vi "xy_graph_coil.vi"() -> ()   [LabVIEW 2019]
panel:
  out "XY Graph":cluster{dbl[], dbl[]}(graph)
  in  "stop":bool
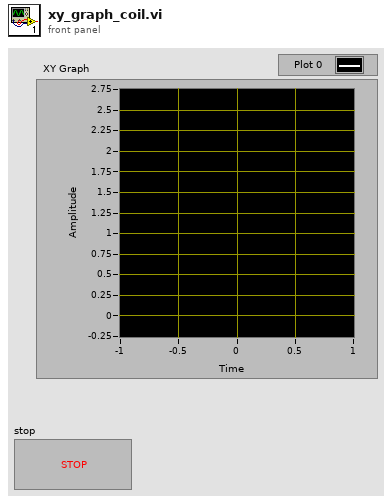
[diagram p1: front panel]
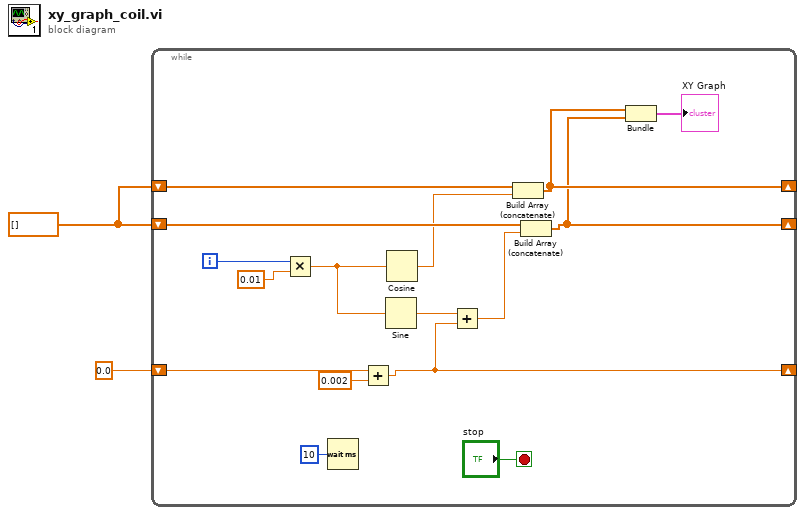
[diagram p0: block diagram]
diagram:
  w2 = dbl[] []
  n1 = while {
    shift-right: [w12] -> _
    shift-left: w2 -> [w16]
    shift-right: [w13] -> _
    shift-left: w2 -> [w15]
    shift-right: [w3] -> _
    shift-left: 0.0 -> [w7]
    i -> [w11]
    stop <- "stop" stop-if-true
    n2 = Multiply(x=w11, y=0.01) -> (x*y=w9:dbl)
    n3 = Wait (ms)(milliseconds to wait=u32 10) -> ()  [unwired: 1 out]
    n4 = Add(x=w7, y=0.002) -> (x+y=w3:dbl)
    n5 = Sine(x=w9) -> (sin(x)=w5:dbl)
    n6 = Cosine(x=w9) -> (cos(x)=w8:dbl)
    n7 = Add(x=w5, y=w3) -> (x+y=w4:dbl)
    n8 = Build Array (concatenate)(w15, w8) -> (w13:dbl[])
    n9 = Build Array (concatenate)(w16, w4) -> (w12:dbl[])
    n10 = Bundle(w13, w12) -> (→"XY Graph":cluster{dbl[], dbl[]})  [unwired: 1 in]
  }
